vi "Start Exiting MHLC.vi"(8 "error in (no error)":errorcluster, 11 "Debug Server in":refnum<class "Debug Server.lvclass">) -> (0 "error out":errorcluster, 3 "Debug Server out":refnum<class "Debug Server.lvclass">)   [LabVIEW 2017, in "Debug Server.lvclass"]
doc: "Get shutdown data from all subWorkers."
uses:
  Debug Server.lvclass
  C:/Program Files (x86)/National Instruments/LabVIEW 2017/vi.lib/addons/_Workers/Library/Classes/Worker/Worker.lvclass
  Settings/rqp_Receive Shutdown Data.ctl
  <vilib>/Utility/miscctls.llb/LVRectTypeDef.ctl
  Debug Server.lvclass/Debug Server.ctl
  Application Manager/Application Manager.lvclass
  Settings/Settings.lvclass
  Message Log/Message Log.lvclass
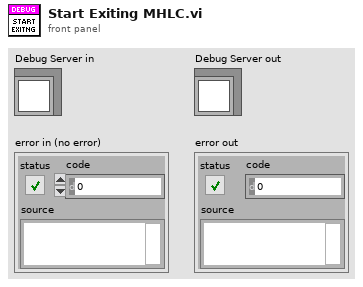
[diagram p1: front panel]
types:
  T1 = typedef "Settings.lvclass/rqp_Receive Shutdown Data.ctl" = cluster{"App Manager":cluster{"WinBounds":T2, "FP.State":enum32{"Invalid", "Standard", "Closed", "Hidden", "Minimized", "Maximized"}, "Monitor":u16, "Column Widths":u32[]}, "Message Log":cluster{"Visible Columns":bool[], "Splitter Position":i32, "Column Widths":u32[], "WinBounds":T2, "FP.State":enum32{"Invalid", "Standard", "Closed", "Hidden", "Minimized", "Maximized"}, "Monitor":u16}}
  T2 = typedef "LVRectTypeDef.ctl" = cluster{"Left":i16, "Top":i16, "Right":i16, "Bottom":i16}
  T3 = typedef "Debug Server.lvclass/Dynamic Message Log Data.ctl" = cluster{"Message Log":refnum<class "Message Log.lvclass">, "DC_UID":T4, "Message Log ID":T5}
  T4 = typedef "DC_UID.ctl" = string
  T5 = typedef "Message Log ID.ctl" = cluster{"Head Worker ID":string, "IP Address":string}
  T6 = enum32{"Invalid", "Standard", "Closed", "Hidden", "Minimized", "Maximized"}
  T7 = typedef "Message Log.lvclass/rwr_Get Shutdown Data Reply.ctl" = cluster{"Config Data":T8}
  T8 = typedef "Message Log.lvclass/Config Data.ctl" = cluster{"Max Num Rows":i32, "Visible Columns":bool[], "Splitter Position":i32, "Column Widths":u32[], "WinBounds":T2, "FP.State":enum32{"Invalid", "Standard", "Closed", "Hidden", "Minimized", "Maximized"}, "Monitor":u16, "Logging":bool, "LogBaseFolder":path}
  T9 = typedef "Application Manager.lvclass/rwr_Get Shutdown Data Reply.ctl" = cluster{"Window Bounds":T2, "Monitor":u16, "FP.State":enum32{"Invalid", "Standard", "Closed", "Hidden", "Minimized", "Maximized"}, "Column Widths":u32[]}
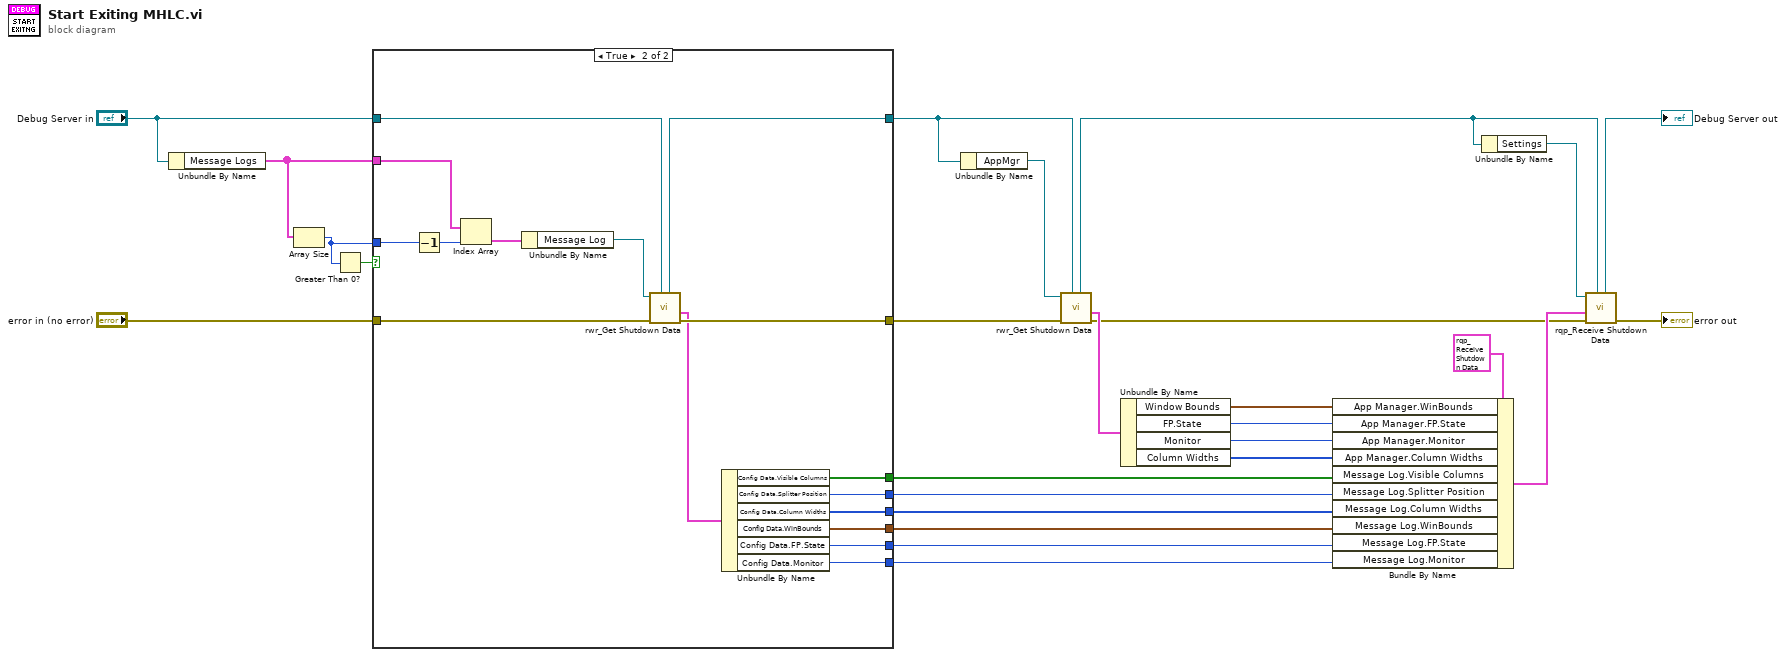
[diagram p0: block diagram]
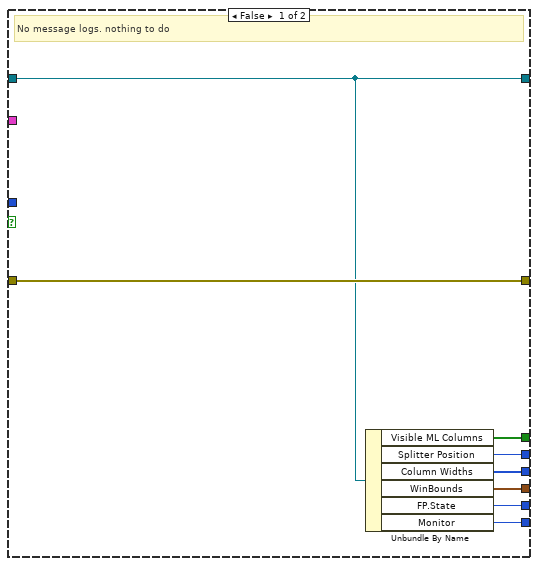
[diagram p2: hidden frame]
diagram:
  n1 = Unbundle By Name("Debug Server in") -> ("Message Logs"=w14:T3[])
  n2 = Array Size(array=w14) -> (size(s)=w9:i32)
  n3 = Greater Than 0?(x=w9) -> (x > 0?=w10:bool)
  n4 = case shown="True" w10 {
    tunnel: "error in (no error)" -> [w34 w50]
    tunnel: w14 -> [_ w49]
    tunnel: [w34 w48] -> w12
    tunnel: "Debug Server in" -> [w33 w47]
    tunnel: [w33 w46] -> w8
    tunnel: w9 -> [_ w42]
    tunnel: [w32 w40] -> w7
    tunnel: [w31 w39] -> w6
    tunnel: [w30 w38] -> w5
    tunnel: [w29 w37] -> w4
    tunnel: [w28 w36] -> w3
    tunnel: [w27 w35] -> w2
    frame False {
      # "No message logs. nothing to do"
      n5 = Unbundle By Name(w33) -> ("Visible ML Columns"=w32:bool[], "Splitter Position"=w31:i32, "Column Widths"=w30:u32[], "WinBounds"=w29:T2, "FP.State"=w28:T6, "Monitor"=w27:u16)
    }
    frame True {
      n6 = Decrement(x=w42) -> (x-1=w43:i32)
      n7 = Index Array(array=w49, index=w43) -> (element=w45:T3)
      n8 = Unbundle By Name(w45) -> ("Message Log"=w44:refnum<class "Message Log.lvclass">)
      n9 = call "rwr_Get Shutdown Data.vi"("Caller in"=w47, "error in"=w50, "Message Log in"=w44) -> ("error out"=w48:errorcluster, "Reply Data out"=w41:T7, "dup Caller out"=w46:refnum<class "Debug Server.lvclass">)  [unwired: 5 in, 1 out]
      n10 = Unbundle By Name(w41) -> ("Config Data.Visible Columns"=w40:bool[], "Config Data.Splitter Position"=w39:i32, "Config Data.Column Widths"=w38:u32[], "Config Data.WinBounds"=w37:T2, "Config Data.FP.State"=w36:T6, "Config Data.Monitor"=w35:u16)
    }
  }
  n11 = Unbundle By Name(w8) -> ("AppMgr"=w13:refnum<class "Application Manager.lvclass">)
  n12 = call "rwr_Get Shutdown Data.vi"("Caller in"=w8, "error in"=w12, "Application Manager in"=w13) -> ("error out"=w17:errorcluster, "Reply Data out"=w22:T9, "dup Caller out"=w1:refnum<class "Debug Server.lvclass">)  [unwired: 5 in, 1 out]
  n13 = Unbundle By Name(w22) -> ("Window Bounds"=w23:T2, "FP.State"=w24:T6, "Monitor"=w25:u16, "Column Widths"=w26:u32[])
  n14 = Bundle By Name(cluster=T1 {"App Manager"={"WinBounds"={"Left"=0, "Top"=0, "Right"=0, "Bottom"=0}, "FP.State"=enum."Invalid", "Monitor"=0, "Column Widths"=[]}, "Message Log"={"Visible Columns"=[], "Splitter Position"=0, "Column Widths"=[], "WinBounds"={"Left"=0, "Top"=0, "Right"=0, "Bottom"=0}, "FP.State"=enum."Invalid", "Monitor"=0}} ("Data in"), "App Manager.WinBounds"=w23, "App Manager.FP.State"=w24, "App Manager.Monitor"=w25, "App Manager.Column Widths"=w26, "Message Log.Visible Columns"=w7, "Message Log.Splitter Position"=w6, "Message Log.Column Widths"=w5, "Message Log.WinBounds"=w4, "Message Log.FP.State"=w3, "Message Log.Monitor"=w2) -> (w21:T1)
  n15 = Unbundle By Name(w1) -> ("Settings"=w19:refnum<class "Settings.lvclass">)
  n16 = call "rqp_Receive Shutdown Data.vi"("Caller in"=w1, "error in"=w17, "Data in"=w21, "Settings in"=w19) -> ("error out"=→"error out":errorcluster, "dup Caller out"=→"Debug Server out":refnum<class "Debug Server.lvclass">)  [unwired: 5 in, 1 out]
